vi "MPM_Logging_Start.vi"(8 "error in (no error)":errorcluster, 11 ".NET Reference in":refnum<k24>) -> (0 "error out":errorcluster, 3 "Reference out":refnum<k24>)   [LabVIEW 2017]
doc: "MPM sampling start"
uses:
  D:/test/ILSTS/LV_IL_Sample/DLL/InstrumentDLL.dll
  DLL/InstrumentDLL.dll
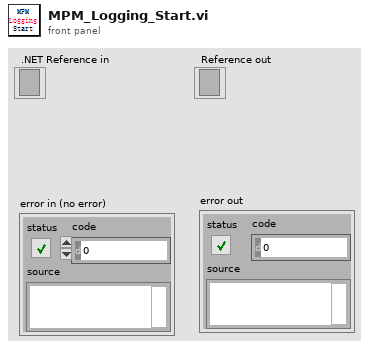
[diagram p1: front panel]
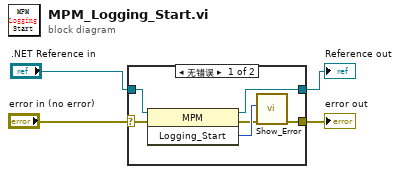
[diagram p0: block diagram]
diagram:
  n1 = case shown="无错误" "error in (no error)" {
    selector: "error in (no error)" -> [w7 w12]
    tunnel: [w8 w12] -> w4
    tunnel: ".NET Reference in" -> [w6 w11]
    tunnel: [w5 w11] -> w1
    frame No Error {
      n2 = invoke class="MPM" method="Logging_Start"(reference=w6, error in=w7) -> (reference out=w5:refnum<k24>, error out=w9:errorcluster, "Logging_Start"=w10:i32)  [unwired: 1 in]
      n3 = call "Show_Error.vi"("error in (no error)"=w9, "Error"=w10) -> ("error out"=w8:errorcluster)  [unwired: 9 in]
    }
    frame Error {
    }
  }
  "Reference out" <- w1
  "error out" <- w4
